vi "HistogramRange (SubVI).vi"(6 "offset":i32, 8 "Histogram Graph3":u32[](graph), 9 "Histogram Graph2":u32[](graph), 10 "Histogram Graph1":u32[](graph)) -> (2 "Output Range":T1)   [LabVIEW 2019]
doc: "c 2020 ReMiSYS All rights reserved."
panel:
  # "c 2020 ReMiSYS All rights reserved."
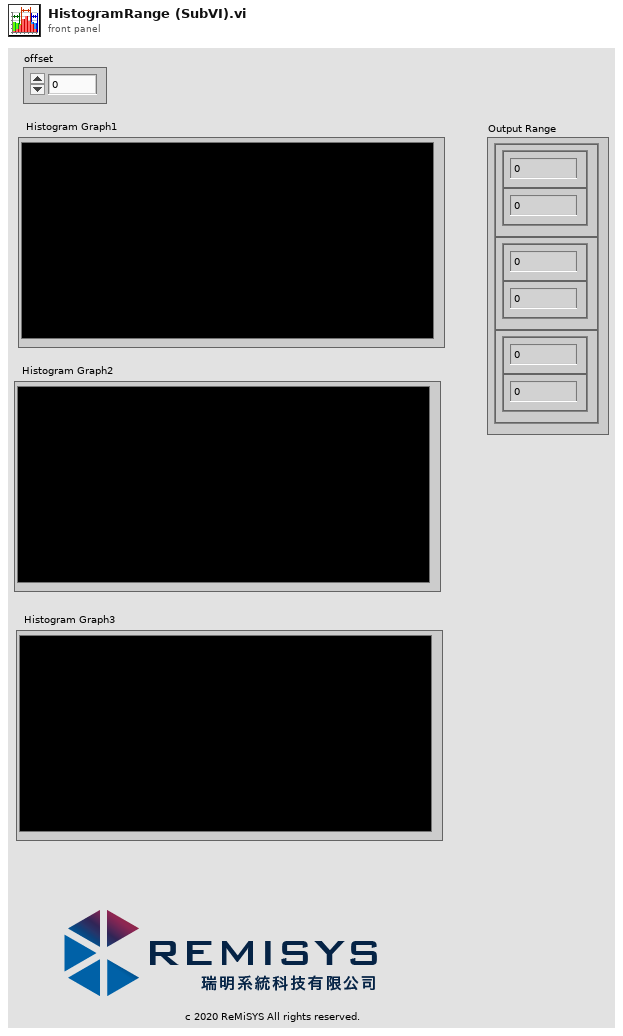
[diagram p1: front panel]
types:
  T1 = cluster{"Cluster":cluster{"Numeric Control":i32, "Numeric Control":i32}, "Cluster":cluster{"Numeric Control":i32, "Numeric Control":i32}, "Cluster":cluster{"Numeric Control":i32, "Numeric Control":i32}}
  T2 = cluster{"Numeric Control":i32, "Numeric Control":i32}
  T3 = cluster{"Output Range":cluster{"Numeric Control":i32, "Numeric Control":i32}, "Output Range":cluster{"Numeric Control":i32, "Numeric Control":i32}, "Output Range":cluster{"Numeric Control":i32, "Numeric Control":i32}}
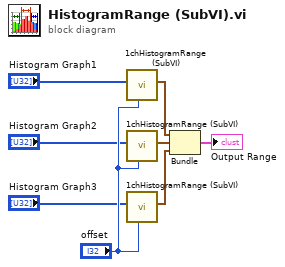
[diagram p0: block diagram]
diagram:
  n1 = call "1chHistogramRange (SubVI).vi"("offset"="offset", "Histogram 1"="Histogram Graph1") -> ("Output Range"=w8:T2)  [unwired: 9 in]
  n2 = call "1chHistogramRange (SubVI).vi"("offset"="offset", "Histogram 1"="Histogram Graph2") -> ("Output Range"=w7:T2)  [unwired: 9 in]
  n3 = call "1chHistogramRange (SubVI).vi"("offset"="offset", "Histogram 1"="Histogram Graph3") -> ("Output Range"=w6:T2)  [unwired: 9 in]
  n4 = Bundle("Output Range"=w8, "Output Range"=w7, "Output Range"=w6) -> (→"Output Range":T3)  [unwired: 1 in]
